vi "Wolna_obliczenia.vi"(5 "Wektor1 in":waveform(dbl), 6 "Typ rejestracji":T1, 7 "Wektor2 in":waveform(dbl), 8 "error in (no error)":errorcluster, 9 "Okres (0,02)":dbl=0.02, 10 "Zakresy":dbl[](array[numeric]), 11 "Wolna in":waveform(dbl)) -> (0 "error out":errorcluster, 2 "Value out":dbl, 3 "Wolna out":waveform(dbl))   [LabVIEW 2014]
doc: "Oblicza operacje na sygnalach\nwolnych"
uses:
  Kontrolki/GUI/RejWol_typ.ctl
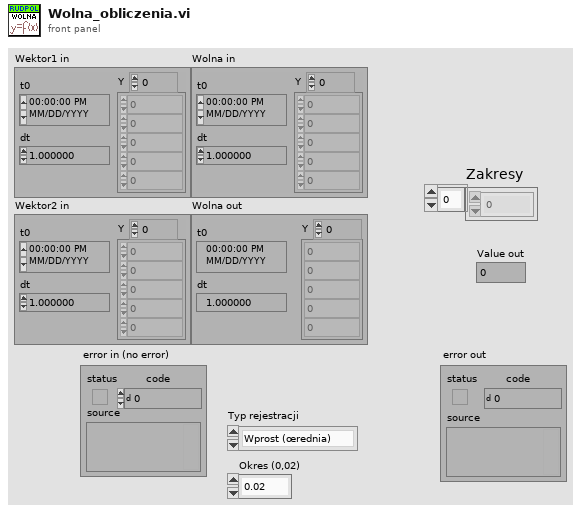
[diagram p1: front panel]
types:
  T1 = typedef "RejWol_typ.ctl" = enum16{"Wprost (œrednia)", "Modu³ (œr. wypr)", "Kwadrat (skuteczna)", "Iloczyn", "Faza"}
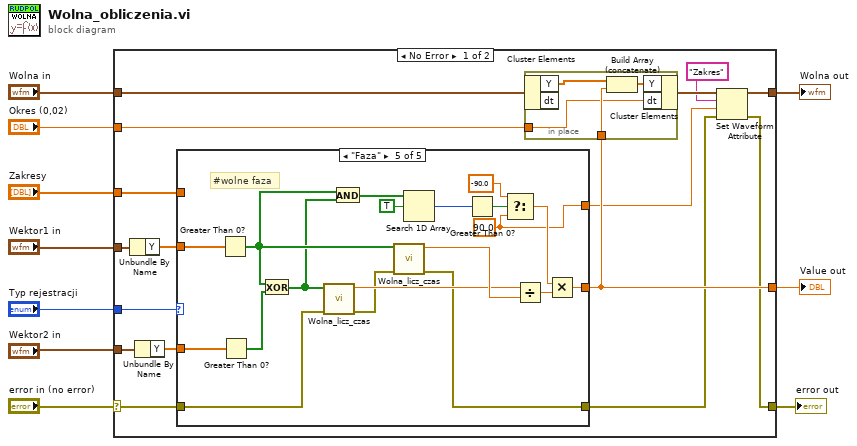
[diagram p0: block diagram]
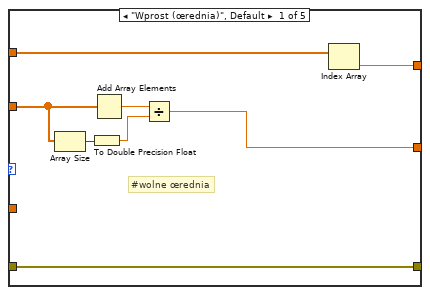
[diagram p2: hidden frame]
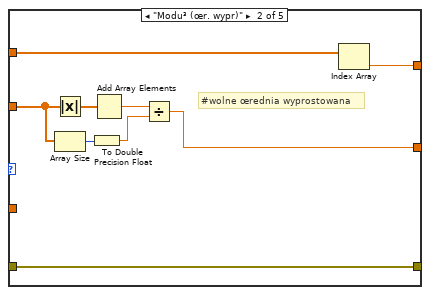
[diagram p3: hidden frame]
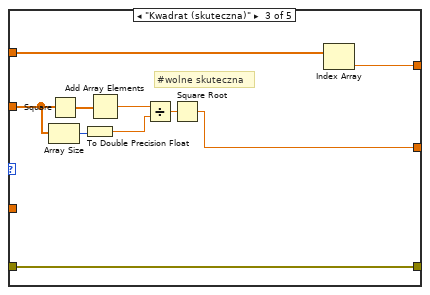
[diagram p4: hidden frame]
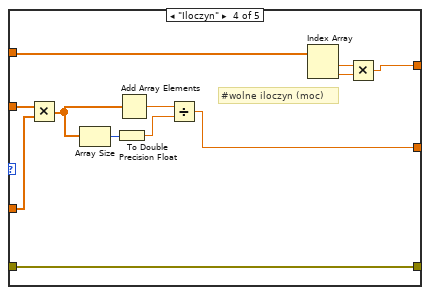
[diagram p5: hidden frame]
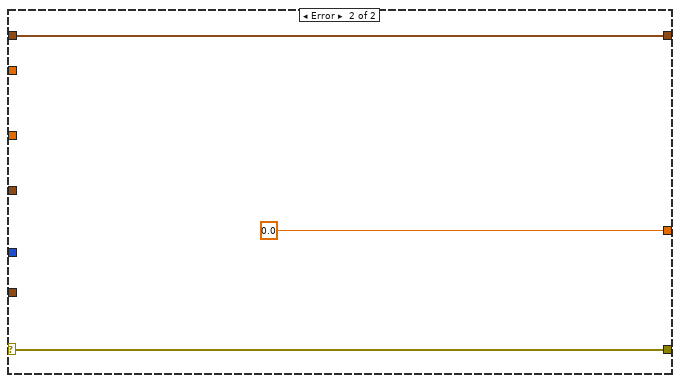
[diagram p6: hidden frame]
diagram:
  n1 = case shown="No Error" "error in (no error)" {
    selector: "error in (no error)" -> [w25 w91]
    tunnel: [w11 w91] -> w9
    tunnel: "Typ rejestracji" -> [w26 _]
    tunnel: [w19 0.0 ("Numeric")] -> w7
    tunnel: "Wektor1 in" -> [w23 _]
    tunnel: "Wektor2 in" -> [w21 _]
    tunnel: "Wolna in" -> [w20 w89]
    tunnel: [w15 w89] -> w3
    tunnel: "Okres (0,02)" -> [w18 _]
    tunnel: "Zakresy" -> [w17 _]
    frame No Error {
      n2 = Unbundle By Name(w23) -> ("Y"=w24:dbl[])
      n3 = Unbundle By Name(w21) -> ("Y"=w22:dbl[])
      n4 = case shown="\"Faza\"" w26 {
        tunnel: w24 -> [w34 w44 w57 w66 w87]
        tunnel: w22 -> [_ _ _ w65 w88]
        tunnel: w25 -> [w38 w42 w51 w63 w75]
        tunnel: [w38 w42 w51 w63 w73] -> w12
        tunnel: [w33 w41 w50 w62 w71] -> w19
        tunnel: w17 -> [w32 w40 w49 w61 _]
        tunnel: [w31 w39 w48 w58 w70] -> w14
        frame "Wprost (œrednia)", Default {
          # "#wolne œrednia"
          n5 = Array Size(array=w34) -> (size(s)=w37:i32)
          n6 = To Double Precision Float(number=w37) -> (double precision float=w35:dbl)
          n7 = Add Array Elements(numeric array=w34) -> (sum=w36:dbl)
          n8 = Divide(x=w36, y=w35) -> (x/y=w33:dbl)
          n9 = Index Array(array=w32) -> (element=w31:dbl)  [unwired: 1 in]
        }
        frame "Modu³ (œr. wypr)" {
          # "#wolne œrednia wyprostowana"
          n10 = Absolute Value(x=w44) -> (abs(x)=w43:dbl[])
          n11 = Array Size(array=w44) -> (size(s)=w47:i32)
          n12 = To Double Precision Float(number=w47) -> (double precision float=w45:dbl)
          n13 = Add Array Elements(numeric array=w43) -> (sum=w46:dbl)
          n14 = Divide(x=w46, y=w45) -> (x/y=w41:dbl)
          n15 = Index Array(array=w40) -> (element=w39:dbl)  [unwired: 1 in]
        }
        frame "Kwadrat (skuteczna)" {
          # "#wolne skuteczna"
          n16 = Array Size(array=w57) -> (size(s)=w55:i32)
          n17 = Square(x=w57) -> (x^2=w56:dbl[])
          n18 = To Double Precision Float(number=w55) -> (double precision float=w53:dbl)
          n19 = Add Array Elements(numeric array=w56) -> (sum=w54:dbl)
          n20 = Divide(x=w54, y=w53) -> (x/y=w52:dbl)
          n21 = Square Root(x=w52) -> (sqrt(x)=w50:dbl)
          n22 = Index Array(array=w49) -> (element=w48:dbl)  [unwired: 1 in]
        }
        frame "Iloczyn" {
          # "#wolne iloczyn (moc)"
          n23 = Multiply(x=w66, y=w65) -> (x*y=w64:dbl[])
          n24 = Array Size(array=w64) -> (size(s)=w69:i32)
          n25 = To Double Precision Float(number=w69) -> (double precision float=w67:dbl)
          n26 = Add Array Elements(numeric array=w64) -> (sum=w68:dbl)
          n27 = Divide(x=w68, y=w67) -> (x/y=w62:dbl)
          n28 = Index Array(array=w61) -> (element #1=w60:dbl, element #2=w59:dbl)  [unwired: 2 in]
          n29 = Multiply(x=w60, y=w59) -> (x*y=w58:dbl)
        }
        frame "Faza" {
          w70 = 90.0
          # "#wolne faza"
          n30 = Greater Than 0?(x=w87) -> (x > 0?=w80:bool[])
          n31 = Greater Than 0?(x=w88) -> (x > 0?=w86:bool[])
          n32 = Exclusive Or(1:w86, 2:w80) -> (0:w72:bool[])
          n33 = call "Wolna_licz_czas.vi"("error in (no error)"=w75, "Array"=w72) -> ("error out"=w74:errorcluster, "l.probek"=w76:dbl)  [unwired: 8 in]
          n34 = And(x=w80, y=w72) -> (x .and. y?=w78:bool[])
          n35 = call "Wolna_licz_czas.vi"("error in (no error)"=w74, "Array"=w80) -> ("error out"=w73:errorcluster, "l.probek"=w85:dbl)  [unwired: 8 in]
          n36 = Search 1D Array(1D array=w78, element=TRUE) -> (index of element=w77:i32)  [unwired: 1 in]
          n37 = Greater Than 0?(x=w77) -> (x > 0?=w82:bool)
          n38 = Select(t=-90.0, s=w82, f=w70) -> (s? t:f=w81:dbl)
          n39 = Divide(x=w76, y=w85) -> (x/y=w84:dbl)
          n40 = Multiply(x=w81, y=w84) -> (x*y=w71:dbl)
        }
      }
      n41 = in-place {
        in-place-border: w19 -> [w28]
        in-place-border: w18 -> [w27]
        n42 = in-place-cluster #1(w20) -> ("Y"=w30:dbl[])  [unwired: 1 out]
        n43 = Build Array (concatenate)(w30, w28) -> (w29:dbl[])
        n44 = in-place-cluster #1("Y"=w29, "dt"=w27) -> (w16:waveform(dbl))
      }
      n45 = Set Waveform Attribute(4:w12, 5:w14, 6:"Zakres" ("name"), 7:w16) -> (0:w11:errorcluster, 3:w15:waveform(dbl))  [unwired: 1 out]
    }
    frame Error {
    }
  }
  "error out" <- w9
  "Value out" <- w7
  "Wolna out" <- w3
